vi "SM motor repeat TDC DS345 tw.vi"(0 "SM Config":T5={"VISA Serial ref"="COM3", "Motor Config"={"DriveRatio (mm/rev)"=10.16, "PosLimit + (mm)"=200.0, "PosLimit - (mm)"=0.0, "EncoderRatio (count/rev)"=2000.0, "MotorType"=enum."SM17"}} {"Motor Config"."EncoderRatio (count/rev)" format="%.2f"; "Motor Config"."PosLimit - (mm)" format="%.3f"; "Motor Config"."PosLimit + (mm)" format="%.3f"; "Motor Config"."DriveRatio (mm/rev)" format="%.2f"}, 1 "Waiting time (s)":dbl=3.0, 5 "SM setting":T4={"Acceleration (mm/sec^2)"=1000.0, "Velocity (mm/sec)"=1.0, "Position (mm)"=0.0} {"Position (mm)" format="%.3f"; "Velocity (mm/sec)" format="%.3f"; "Acceleration (mm/sec^2)" format="%.3f"}, 7 "Serial":i32=83858441, 9 "Move":bool, 11 "Stop motion":bool, 12 "Moving times":dbl, 13 "Moving parameters":T2={"Velocity (mm/s)"=0.5, "Abs position (mm)"=0.0, "Lasting time (s)"=25.0}) -> (4 "Position (mm)":dbl, 10 "Status":T3)   [LabVIEW 2015]
uses:
  magnetometers/smi/labview/CPM20Software/SmartMotor.llb/SM Config.ctl
  magnetometers/smi/labview/CPM20Software/SmartMotor.llb/SM MotorConfig.ctl
  magnetometers/smi/labview/CPM20Software/SmartMotor.llb/SM Status.ctl
  Global vab.vi
panel:
  in  "stop":bool
  out "Status (s)":dbl
  in  "Lasting time (s)":dbl=10.0
  in  "Default setting (DS345)":T1={"Osc. Amp. (V)"=0.01, "Osc. Freq. (Hz)"=1000.0} {"Osc. Freq. (Hz)" min=0.001 max=250000.0 step=0.001 format="%.3f"; "Osc. Amp. (V)" min=0.0 max=0.1 step=0.001 format="%.3f"}
  in  "Cluster":T1={"Osc. Amp. (V)"=0.06, "Osc. Freq. (Hz)"=1200.0} {"Osc. Freq. (Hz)" min=0.001 max=250000.0 step=0.001 format="%.3f"; "Osc. Amp. (V)" min=0.0 max=10.0 step=0.001 format="%.3f"}
  in  "SRS DS345 GPIB address":string="0:18"
  out "Ccurrent times":dbl
  in  "Action":bool
  # "SM motor setting"
  # "TDC001 motor information"
  # "DS345 information"
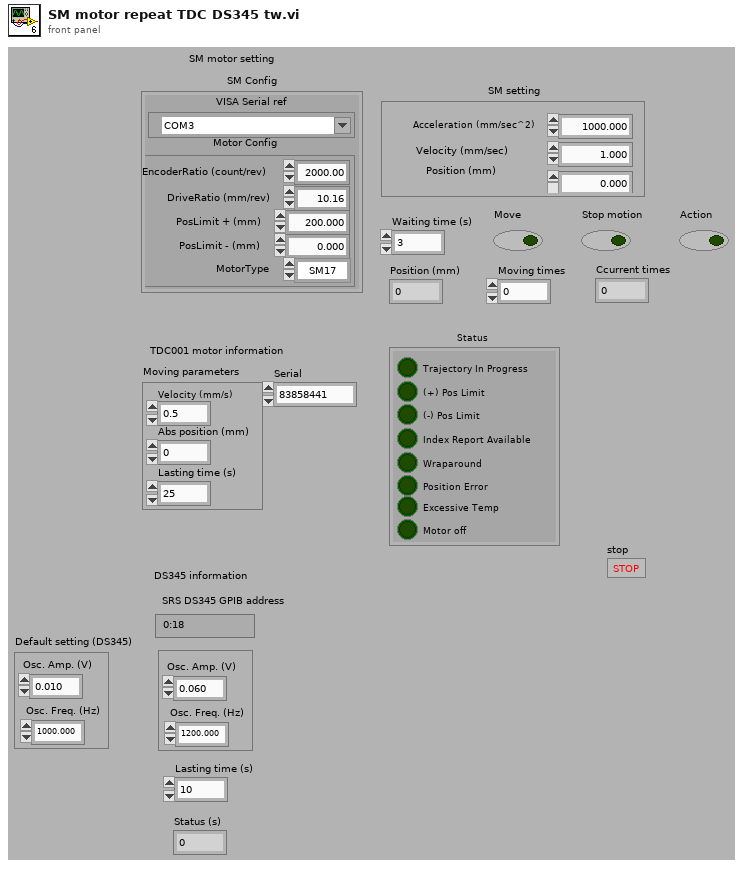
[diagram p1: front panel]
types:
  T1 = cluster{"Osc. Amp. (V)":dbl, "Osc. Freq. (Hz)":dbl}
  T2 = cluster{"Velocity (mm/s)":dbl, "Abs position (mm)":dbl, "Lasting time (s)":dbl}
  T3 = typedef "SM Status.ctl" = cluster{"Trajectory In Progress":bool, "(+) Pos Limit":bool, "(-) Pos Limit":bool, "Index Report Available":bool, "Wraparound":bool, "Position Error":bool, "Excessive Temp":bool, "Motor off":bool}
  T4 = cluster{"Acceleration (mm/sec^2)":dbl, "Velocity (mm/sec)":dbl, "Position (mm)":dbl}
  T5 = typedef "SM Config.ctl" = cluster{"VISA Serial ref":refnum<visa-resource-name>, "Motor Config":T6}
  T6 = typedef "SM MotorConfig.ctl" = cluster{"DriveRatio (mm/rev)":dbl, "PosLimit + (mm)":dbl, "PosLimit - (mm)":dbl, "EncoderRatio (count/rev)":dbl, "MotorType":enum16{"SM17", "SM23", "SM34", "SM42", "SM56"}}
  T7 = cluster{"Acceleration (mm/sec^2)":dbl, "Velocity (mm/sec)":dbl, "PosLimit - (mm)":dbl}
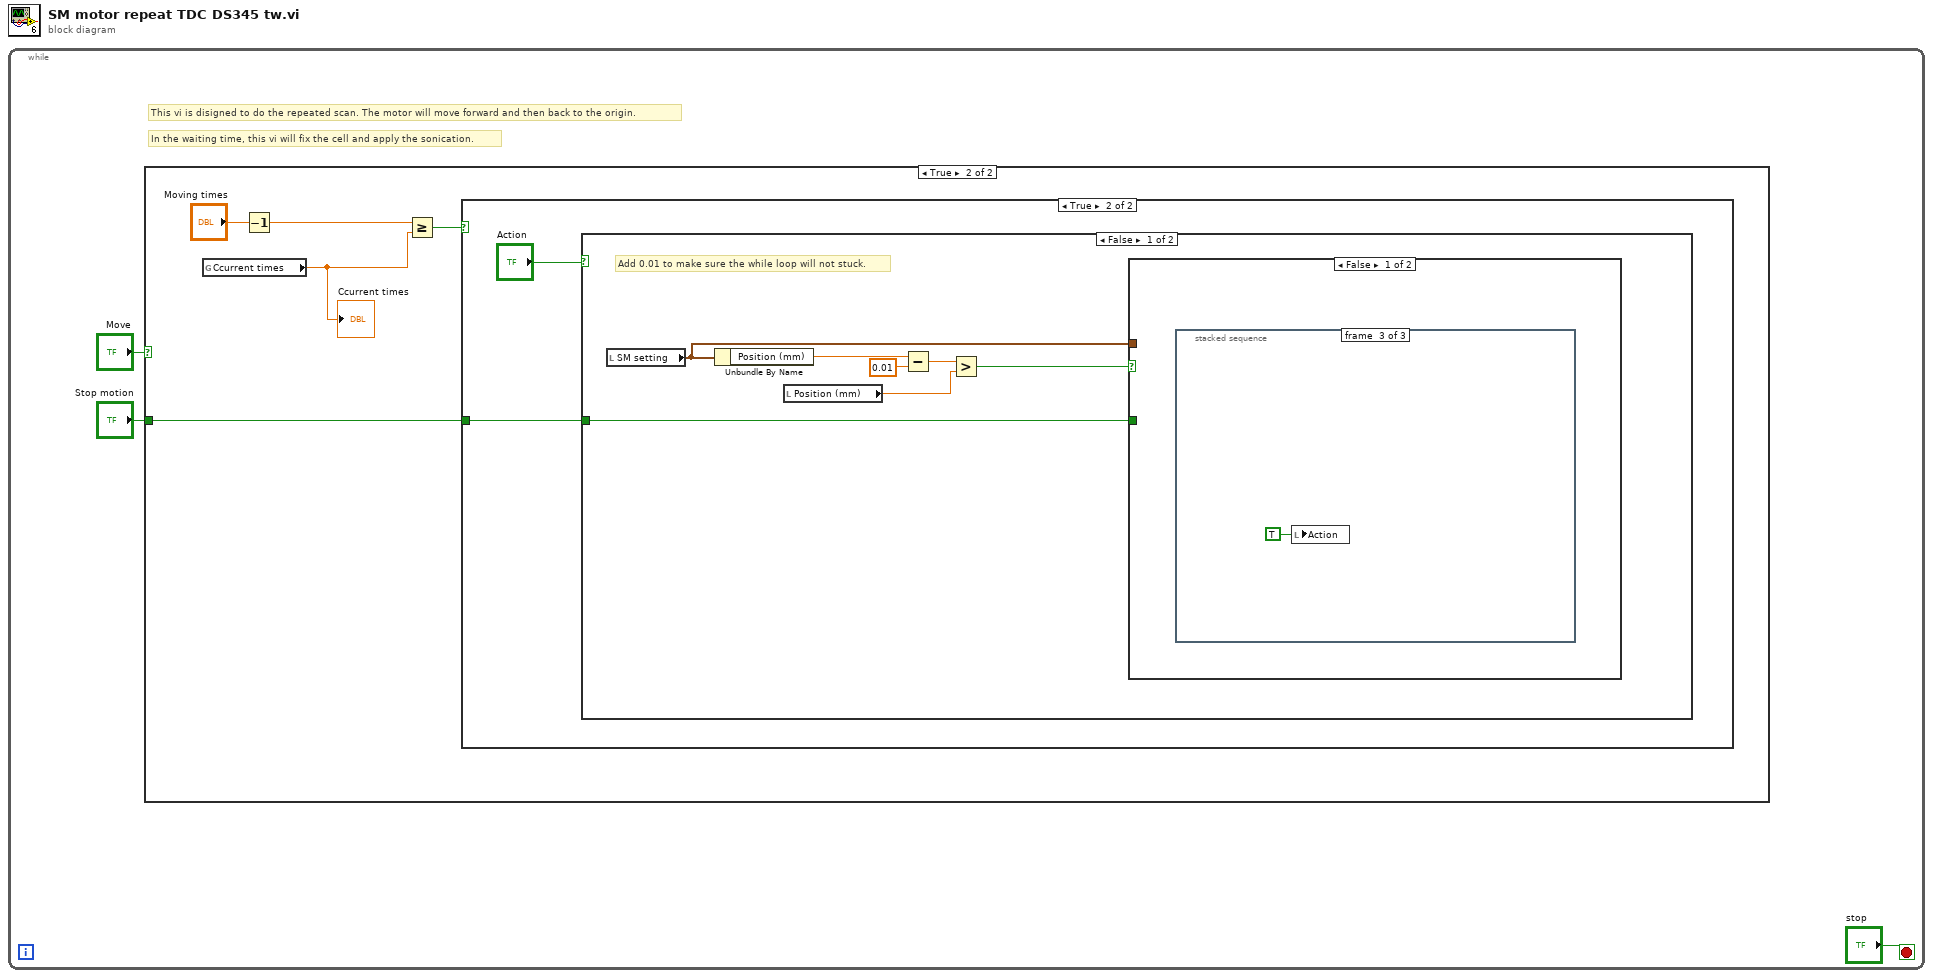
[diagram p0: block diagram]
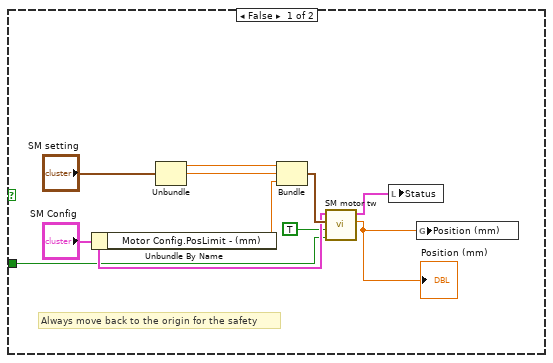
[diagram p2: hidden frame]
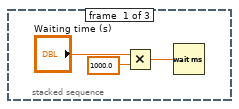
[diagram p4: hidden frame]
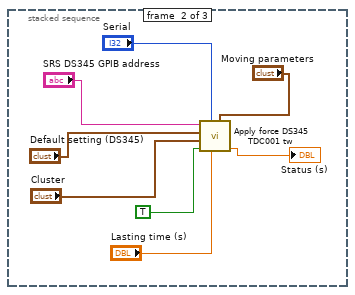
[diagram p5: hidden frame]
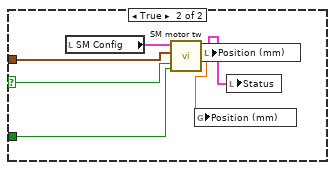
[diagram p6: hidden frame]
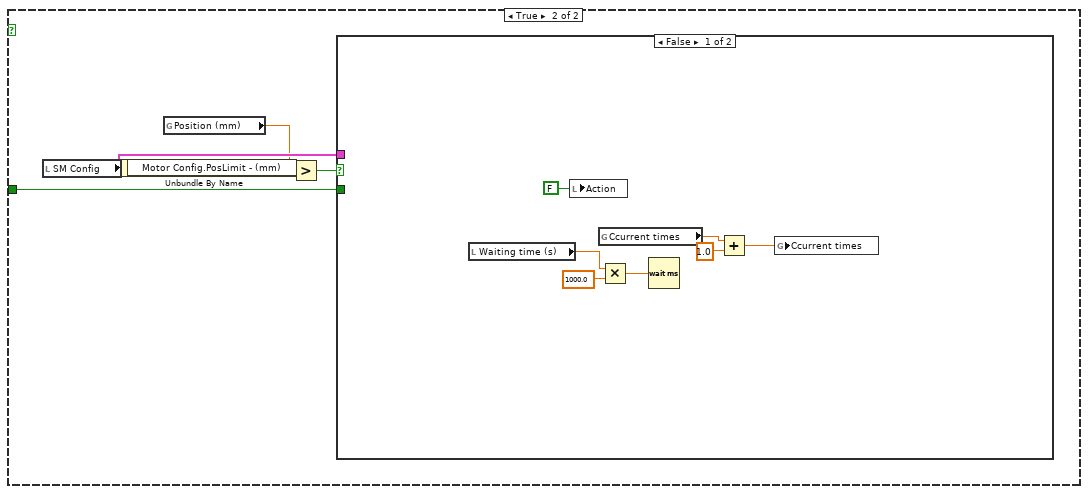
[diagram p7: hidden frame]
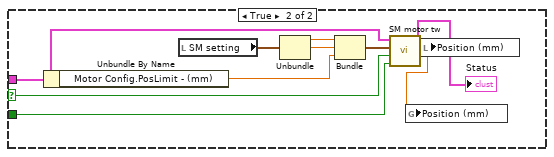
[diagram p8: hidden frame]
diagram:
  n1 = while {
    stop <- "stop" stop-if-true
    # "In the waiting time, this vi will fix the cell and apply the sonication."
    # "This vi is disigned to do the repeated scan. The motor will move forward and then back to the origin."
    n2 = case shown="True" "Move" {
      tunnel: "Stop motion" -> [w6 w16]
      frame False {
        # "Always move back to the origin for the safety"
        n3 = Unbundle By Name("SM Config") -> ("Motor Config.PosLimit - (mm)"=w10:dbl)
        n4 = Unbundle("SM setting") -> ("Acceleration (mm/sec^2)"=w13:dbl, "Velocity (mm/sec)"=w12:dbl)  [unwired: 1 out]
        n5 = Bundle("Acceleration (mm/sec^2)"=w13, "Velocity (mm/sec)"=w12, "PosLimit - (mm)"=w10) -> (w11:T7)  [unwired: 1 out]
        n6 = call "SM motor tw.vi"("SM Config"="SM Config", "SM setting"=w11, "Move"=TRUE, "Stop motion"=w6) -> ("Status"=w4:T3, "Position (mm)"=w5:dbl)  [unwired: 5 out]
        "Position (mm)" <- w5
        n7 = local write "Status"(w4) -> ()
        n8 = global write "Global vab.vi" "Position (mm)"(w5) -> ()
      }
      frame True {
        n9 = global read "Global vab.vi" "Ccurrent times"() -> (w14:dbl)
        "Ccurrent times" <- w14
        n10 = Decrement(x="Moving times") -> (x-1=w15:dbl)
        n11 = Greater Or Equal?(x=w15, y=w14) -> (x >= y?=w17:bool)
        n12 = case shown="True" w17 {
          tunnel: w16 -> [_ w20]
          frame False {
          }
          frame True {
            n13 = case shown="False" "Action" {
              tunnel: w20 -> [w22 w47]
              frame False {
                # "Add 0.01 to make sure the while loop will not stuck."
                n14 = local read "SM setting"() -> (w23:T4)
                n15 = Unbundle By Name(w23) -> ("Position (mm)"=w26:dbl)
                n16 = local read "Position (mm)"() -> (w21:dbl)
                n17 = Subtract(x=w26, y=0.01) -> (x-y=w25:dbl)
                n18 = Greater?(x=w25, y=w21) -> (0:w24:bool)
                n19 = case shown="False" w24 {
                  selector: w24 -> [_ w43]
                  tunnel: w23 -> [_ w44]
                  tunnel: w22 -> [_ w42]
                  frame False {
                    n20 = stacked-sequence {
                      frame #0 {
                        n21 = Multiply(x="Waiting time (s)", y=1000.0) -> (x*y=w30:dbl)
                        n22 = Wait (ms)(milliseconds to wait=w30) -> ()  [unwired: 1 out]
                      }
                      frame #1 {
                        n23 = call "Apply force DS345 TDC001 tw.vi"("Moving parameters"="Moving parameters", "Lasting time (s)"="Lasting time (s)", "TDC001 motor Serial"="Serial", "Apply force"=TRUE, "Cluster"="Cluster", "Default setting (DS345)"="Default setting (DS345)", "SRS DS345 GPIB address"="SRS DS345 GPIB address") -> ("Status (s)"=→"Status (s)":dbl)  [unwired: 3 in]
                      }
                      frame #2 {
                        n24 = local write "Action"(TRUE ("Action")) -> ()
                      }
                    }
                  }
                  frame True {
                    n25 = local read "SM Config"() -> (w45:T5)
                    n26 = call "SM motor tw.vi"("SM Config"=w45, "SM setting"=w44, "Move"=w43, "Stop motion"=w42) -> ("Status"=w40:T3, "Position (mm)"=w41:dbl)  [unwired: 5 out]
                    n27 = global write "Global vab.vi" "Position (mm)"(w41) -> ()
                    n28 = local write "Position (mm)"(w41) -> ()
                    n29 = local write "Status"(w40) -> ()
                  }
                }
              }
              frame True {
                n30 = local read "SM Config"() -> (w49:T5)
                n31 = Unbundle By Name(w49) -> ("Motor Config.PosLimit - (mm)"=w48:dbl)
                n32 = global read "Global vab.vi" "Position (mm)"() -> (w46:dbl)
                n33 = Greater?(x=w46, y=w48) -> (0:w50:bool)
                n34 = case shown="False" w50 {
                  selector: w50 -> [_ w62]
                  tunnel: w49 -> [_ w61]
                  tunnel: w47 -> [_ w60]
                  frame False {
                    n35 = local read "Waiting time (s)"() -> (w52:dbl)
                    n36 = local write "Action"(FALSE ("Action")) -> ()
                    n37 = global read "Global vab.vi" "Ccurrent times"() -> (w55:dbl)
                    n38 = Multiply(x=w52, y=1000.0) -> (x*y=w53:dbl)
                    n39 = Wait (ms)(milliseconds to wait=w53) -> ()  [unwired: 1 out]
                    n40 = Add(x=w55, y=1.0) -> (x+y=w56:dbl)
                    n41 = global write "Global vab.vi" "Ccurrent times"(w56) -> ()
                  }
                  frame True {
                    n42 = Unbundle By Name(w61) -> ("Motor Config.PosLimit - (mm)"=w66:dbl)
                    n43 = local read "SM setting"() -> (w63:T4)
                    n44 = Unbundle(w63) -> ("Acceleration (mm/sec^2)"=w64:dbl, "Velocity (mm/sec)"=w65:dbl)  [unwired: 1 out]
                    n45 = Bundle("Acceleration (mm/sec^2)"=w64, "Velocity (mm/sec)"=w65, "PosLimit - (mm)"=w66) -> (w67:T7)  [unwired: 1 out]
                    n46 = call "SM motor tw.vi"("SM Config"=w61, "SM setting"=w67, "Move"=w62, "Stop motion"=w60) -> ("Status"=→"Status":T3, "Position (mm)"=w59:dbl)  [unwired: 5 out]
                    n47 = global write "Global vab.vi" "Position (mm)"(w59) -> ()
                    n48 = local write "Position (mm)"(w59) -> ()
                  }
                }
              }
            }
          }
        }
      }
    }
  }
